vi "Untitled 1.vi"(9 "clk (B_DIO1 (Pin 13))":bool, 10 "latch (B_DIO2 (Pin 15))":bool, 11 "data (B_DIO0 (Pin 11))":bool) -> (3 "16bit integer":i16)   [LabVIEW 2016]
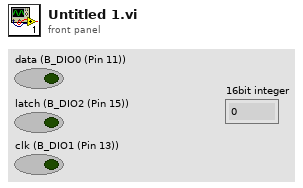
[diagram p1: front panel]
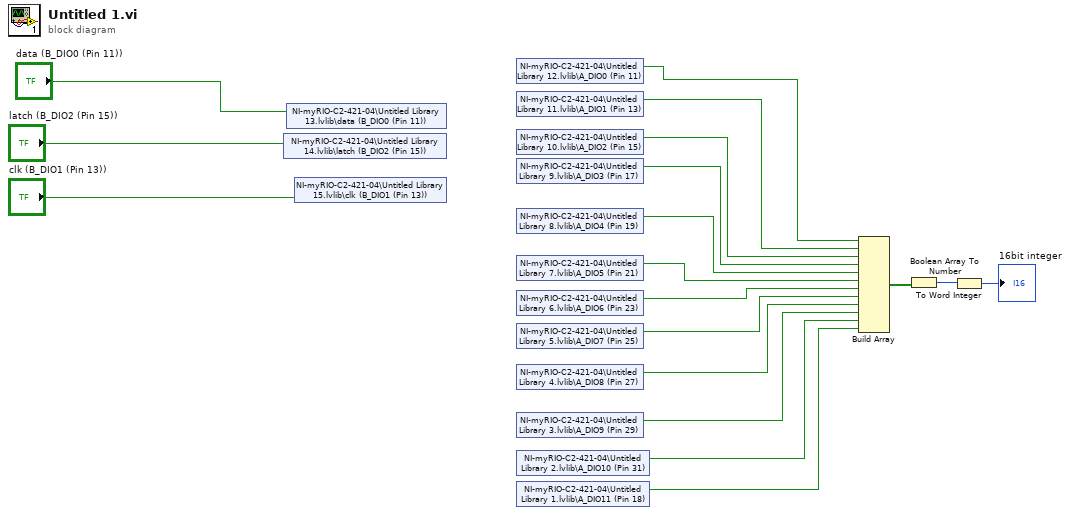
[diagram p0: block diagram]
diagram:
  n1 = shared-variable "NI-myRIO-C2-421-04\\Untitled Library 14.lvlib\\latch (B_DIO2 (Pin 15))"("latch (B_DIO2 (Pin 15))") -> ()  [unwired: 1 in, 1 out]
  n2 = shared-variable "NI-myRIO-C2-421-04\\Untitled Library 13.lvlib\\data (B_DIO0 (Pin 11))"("data (B_DIO0 (Pin 11))") -> ()  [unwired: 1 in, 1 out]
  n3 = shared-variable "NI-myRIO-C2-421-04\\Untitled Library 15.lvlib\\clk (B_DIO1 (Pin 13))"("clk (B_DIO1 (Pin 13))") -> ()  [unwired: 1 in, 1 out]
  n4 = shared-variable "NI-myRIO-C2-421-04\\Untitled Library 12.lvlib\\A_DIO0 (Pin 11)"() -> (w11:bool)  [unwired: 1 in, 1 out]
  n5 = shared-variable "NI-myRIO-C2-421-04\\Untitled Library 11.lvlib\\A_DIO1 (Pin 13)"() -> (w12:bool)  [unwired: 1 in, 1 out]
  n6 = shared-variable "NI-myRIO-C2-421-04\\Untitled Library 10.lvlib\\A_DIO2 (Pin 15)"() -> (w10:bool)  [unwired: 1 in, 1 out]
  n7 = shared-variable "NI-myRIO-C2-421-04\\Untitled Library 9.lvlib\\A_DIO3 (Pin 17)"() -> (w9:bool)  [unwired: 1 in, 1 out]
  n8 = shared-variable "NI-myRIO-C2-421-04\\Untitled Library 8.lvlib\\A_DIO4 (Pin 19)"() -> (w8:bool)  [unwired: 1 in, 1 out]
  n9 = shared-variable "NI-myRIO-C2-421-04\\Untitled Library 7.lvlib\\A_DIO5 (Pin 21)"() -> (w7:bool)  [unwired: 1 in, 1 out]
  n10 = shared-variable "NI-myRIO-C2-421-04\\Untitled Library 6.lvlib\\A_DIO6 (Pin 23)"() -> (w6:bool)  [unwired: 1 in, 1 out]
  n11 = shared-variable "NI-myRIO-C2-421-04\\Untitled Library 5.lvlib\\A_DIO7 (Pin 25)"() -> (w5:bool)  [unwired: 1 in, 1 out]
  n12 = shared-variable "NI-myRIO-C2-421-04\\Untitled Library 4.lvlib\\A_DIO8 (Pin 27)"() -> (w4:bool)  [unwired: 1 in, 1 out]
  n13 = shared-variable "NI-myRIO-C2-421-04\\Untitled Library 3.lvlib\\A_DIO9 (Pin 29)"() -> (w3:bool)  [unwired: 1 in, 1 out]
  n14 = shared-variable "NI-myRIO-C2-421-04\\Untitled Library 2.lvlib\\A_DIO10 (Pin 31)"() -> (w1:bool)  [unwired: 1 in, 1 out]
  n15 = shared-variable "NI-myRIO-C2-421-04\\Untitled Library 1.lvlib\\A_DIO11 (Pin 18)"() -> (w2:bool)  [unwired: 1 in, 1 out]
  n16 = Build Array(w11, w12, w10, w9, w8, w7, w6, w5, w4, w3, w1, w2) -> (w15:bool[])
  n17 = Boolean Array To Number(Boolean array=w15) -> (number=w14:u32)
  n18 = To Word Integer(number=w14) -> (16bit integer=→"16bit integer":i16)
